vi "Read_Lux.vi"(9 "error in (no error)":errorcluster) -> (0 "error out":errorcluster, 1 "Lux_Value":string, 2 "ReadData":string)   [LabVIEW 2017]
panel:
  out "standard error":string
  out "return code":i32
  out "standard output":string
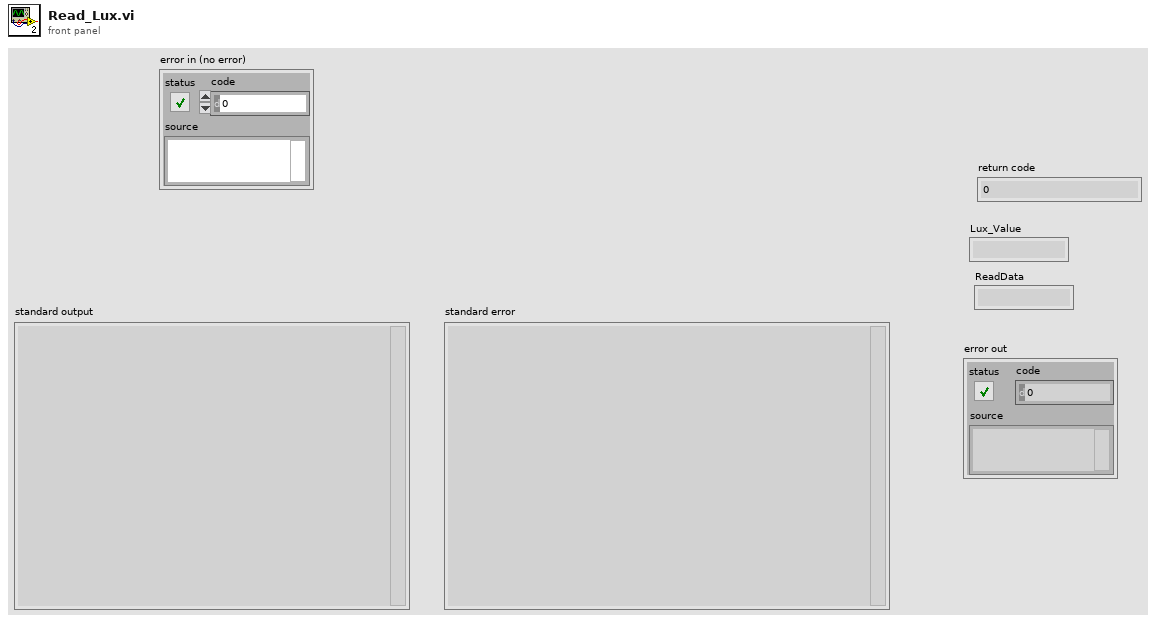
[diagram p1: front panel]
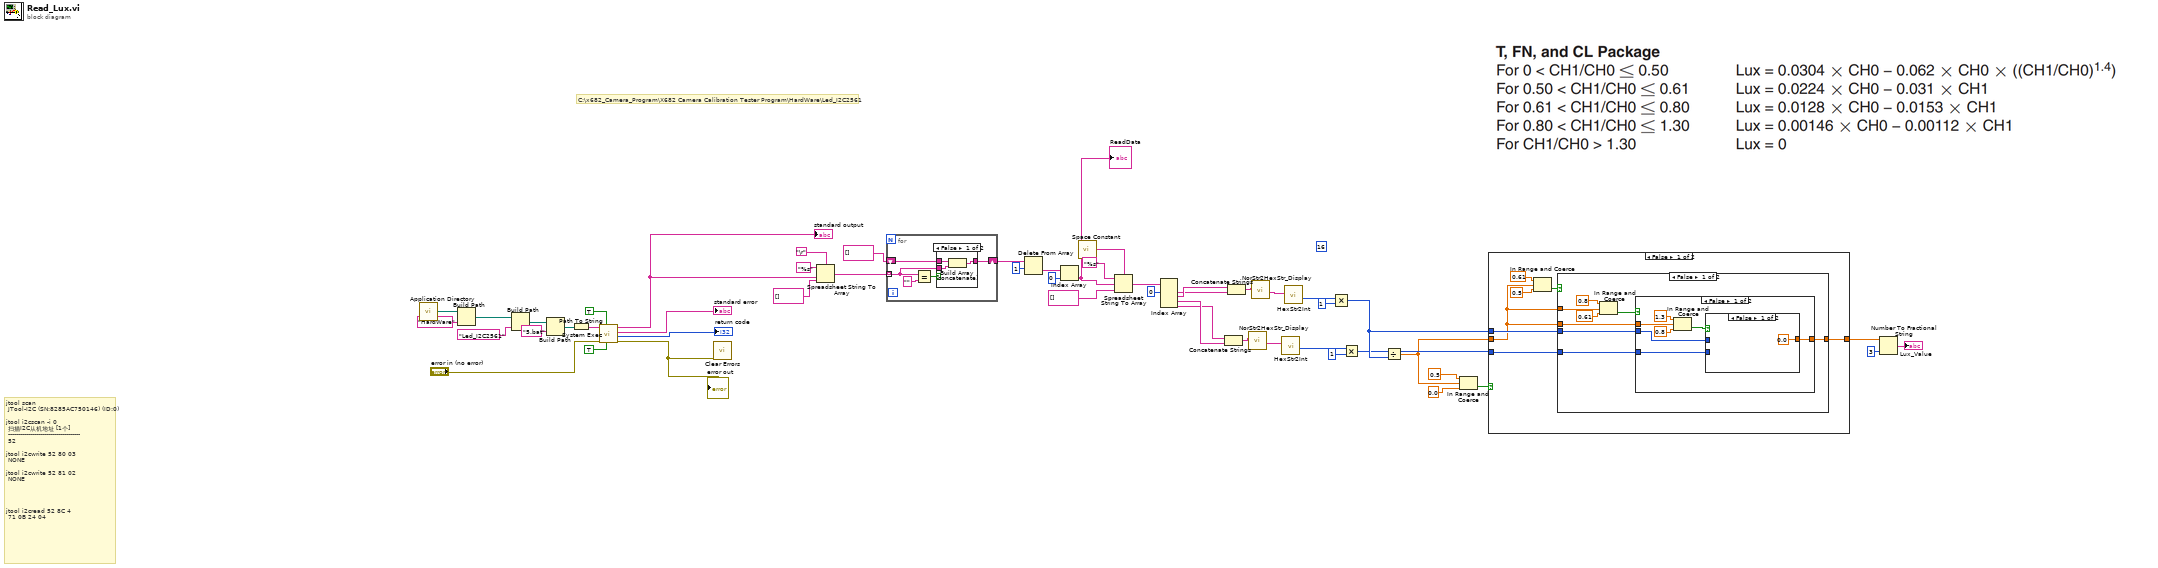
[diagram p0: block diagram]
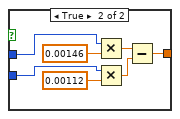
[diagram p2: hidden frame]
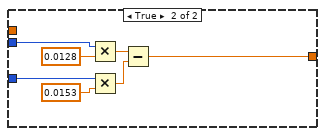
[diagram p3: hidden frame]
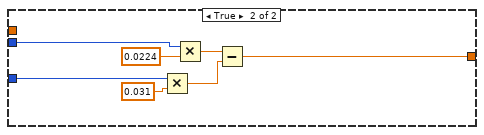
[diagram p4: hidden frame]
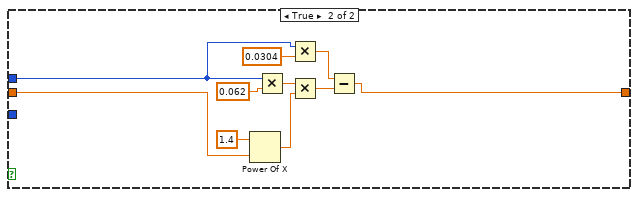
[diagram p5: hidden frame]
diagram:
  (unwired) u32 16 ("y")
  # "C:\\x682_Camera_Program\\X682 Camera Calibration Tester Program\\HardWare\\Led_I2C2561"
  # "jtool scan\n\tJTool-I2C (SN:8285AC750146) (ID:0)\n\t\njtool i2cscan -i 0\n\t扫描I2C从机地址 [1个]\n\t------------------------------------\n\t52\t\n\t\njtool i2cwrite 52 80 03\n\tNONE\n\njtool i2cwrite 52 81 02\t\n\tNONE\n\n\n\n\njtool i2cread 52 8C 4\n\t71 0B 24 04"
  n1 = call <vilib>:"Application Directory.vi"() -> ("Application Directory"=w12:path)
  n2 = Build Path(base path=w12, name or relative path="HardWare") -> (appended path=w10:path)
  n3 = Build Path(base path=w10, name or relative path="Led_I2C2561") -> (appended path=w8:path)
  n4 = Build Path(base path=w8, name or relative path="5.bat") -> (appended path=w6:path)
  n5 = Path To String(path=w6) -> (string=w5:string)
  n6 = call <vilib>:"System Exec.vi"("run minimized? (F)"=TRUE, "wait until completion? (T)"=TRUE, "error in (no error)"="error in (no error)", "command line"=w5) -> ("error out"=w14:errorcluster, "return code"=→"return code":i32, "standard error"=→"standard error":string, "standard output"=w13:string)  [unwired: 2 in, 2 out]
  "standard output" <- w13
  "error out" <- w14
  n7 = call <vilib>:"Clear Errors.vi"("error in (no error)"=w14) -> ()  [unwired: 5 in, 2 out]
  n8 = Spreadsheet String To Array(delimiter (Tab)="\r", format string="%s" ("格式字符串"), spreadsheet string=w13, array type (2D Dbl)=string[] [] ("数组类型(2D Dbl)")) -> (array=w44:string[])
  n9 = for {
    tunnel: w44 -> [w53] mode=indexing
    shift-right: [w52] -> w42
    shift-left: string[] [] -> [w54]
    n10 = Equal?(x=w53, y="") -> (x = y?=w55:bool)
    n11 = case shown="False" w55 {
      tunnel: w54 -> [w59 w60]
      tunnel: w53 -> [w58 _]
      tunnel: [w57 w60] -> w52
      frame False {
        n12 = Build Array (concatenate)(w59, w58) -> (w57:string[])
      }
      frame True {
      }
    }
  }
  n13 = Delete From Array(array=w42, length=1 ("长度")) -> (deleted portion=w40:string[])  [unwired: 1 in, 1 out]
  n14 = Index Array(array=w40, index=0 ("索引")) -> (element=w38:string)
  "ReadData" <- w38
  n15 = call <vilib>:"Space Constant.vi"() -> ("String"=w36:string)
  n16 = Spreadsheet String To Array(delimiter (Tab)=w36, format string="%s" ("格式字符串"), spreadsheet string=w38, array type (2D Dbl)=string[] []) -> (array=w33:string[])
  n17 = Index Array(array=w33, index #1=0 ("索引")) -> (element #1=w30:string, element #2=w31:string, element #3=w26:string, element #4=w25:string)  [unwired: 3 in]
  n18 = Concatenate Strings(w25, w26) -> (w28:string)
  n19 = Concatenate Strings(w31, w30) -> (w29:string)
  n20 = call "NorStr2HexStr_Display.vi"("Normal Display"=w28) -> ("Hex Display"=w27:string)  [unwired: 10 in]
  n21 = call "NorStr2HexStr_Display.vi"("Normal Display"=w29) -> ("Hex Display"=w34:string)  [unwired: 10 in]
  n22 = call "HexStr2Int.vi"("十六进制字符串"=w27) -> ("数字"=w21:u32)  [unwired: 10 in]
  n23 = call "HexStr2Int.vi"("十六进制字符串"=w34) -> ("数字"=w24:u32)  [unwired: 10 in]
  n24 = Multiply(x=w24, y=u32 1) -> (x*y=w19:u32)
  n25 = Multiply(x=w21, y=u32 1) -> (x*y=w18:u32)
  n26 = Divide(x=w18, y=w19) -> (x/y=w17:dbl)
  n27 = In Range and Coerce(upper limit=0.5 ("下限"), x=w17, lower limit=0.0 ("上限")) -> (In Range?=w20:bool)  [unwired: 1 out]
  n28 = case shown="False" w20 {
    tunnel: w19 -> [w66 w111]
    tunnel: w17 -> [w61 w106]
    tunnel: [w64 w107] -> w4
    tunnel: w18 -> [w65 _]
    frame False {
      n29 = In Range and Coerce(upper limit=0.61 ("下限"), x=w61, lower limit=0.5 ("上限")) -> (In Range?=w67:bool)  [unwired: 1 out]
      n30 = case shown="False" w67 {
        tunnel: w66 -> [w73 w103]
        tunnel: w65 -> [w72 w101]
        tunnel: [w71 w98] -> w64
        tunnel: w61 -> [w75 _]
        tunnel: w61 -> [w70 _]
        frame False {
          n31 = In Range and Coerce(upper limit=0.8 ("下限"), x=w75, lower limit=0.61 ("上限")) -> (In Range?=w74:bool)  [unwired: 1 out]
          n32 = case shown="False" w74 {
            tunnel: w73 -> [w80 w95]
            tunnel: w72 -> [w79 w94]
            tunnel: [w78 w91] -> w71
            tunnel: w70 -> [w82 _]
            frame False {
              n33 = In Range and Coerce(upper limit=1.3 ("下限"), x=w82, lower limit=0.8 ("上限")) -> (In Range?=w81:bool)  [unwired: 1 out]
              n34 = case shown="False" w81 {
                tunnel: w80 -> [_ w88]
                tunnel: w79 -> [_ w87]
                tunnel: [0.0 w84] -> w78
                frame False {
                }
                frame True {
                  n35 = Multiply(x=w88, y=0.00146 ("下限")) -> (x*y=w86:dbl)
                  n36 = Multiply(x=w87, y=0.00112 ("下限")) -> (x*y=w85:dbl)
                  n37 = Subtract(x=w86, y=w85) -> (x-y=w84:dbl)
                }
              }
            }
            frame True {
              n38 = Multiply(x=w95, y=0.0128 ("下限")) -> (x*y=w93:dbl)
              n39 = Multiply(x=w94, y=0.0153 ("下限")) -> (x*y=w92:dbl)
              n40 = Subtract(x=w93, y=w92) -> (x-y=w91:dbl)
            }
          }
        }
        frame True {
          n41 = Multiply(x=w101, y=0.031 ("下限")) -> (x*y=w99:dbl)
          n42 = Multiply(x=w103, y=0.0224 ("下限")) -> (x*y=w100:dbl)
          n43 = Subtract(x=w100, y=w99) -> (x-y=w98:dbl)
        }
      }
    }
    frame True {
      n44 = Power Of X(1:w106, 2:1.4 ("x")) -> (0:w109:dbl)
      n45 = Multiply(x=w111, y=0.062 ("下限")) -> (x*y=w110:dbl)
      n46 = Multiply(x=w111, y=0.0304 ("下限")) -> (x*y=w113:dbl)
      n47 = Multiply(x=w110, y=w109) -> (x*y=w108:dbl)
      n48 = Subtract(x=w113, y=w108) -> (x-y=w107:dbl)
    }
  }
  n49 = Number To Fractional String(number=w4, precision (6)=i16 3) -> (F-format string=→"Lux_Value":string)  [unwired: 2 in]
